vi "SR830Test.vi"() -> ()   [LabVIEW 2013]
uses:
  <vilib>/Instr/_visa.llb/VISA Configure Serial Port (Instr).vi
panel:
  out "read buffer":string
  in  "VISA resource name":refnum<visa-resource-name>
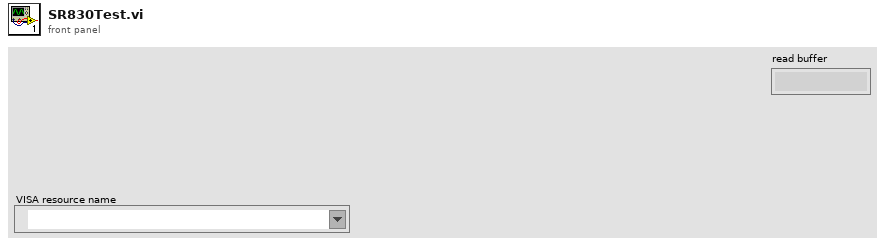
[diagram p1: front panel]
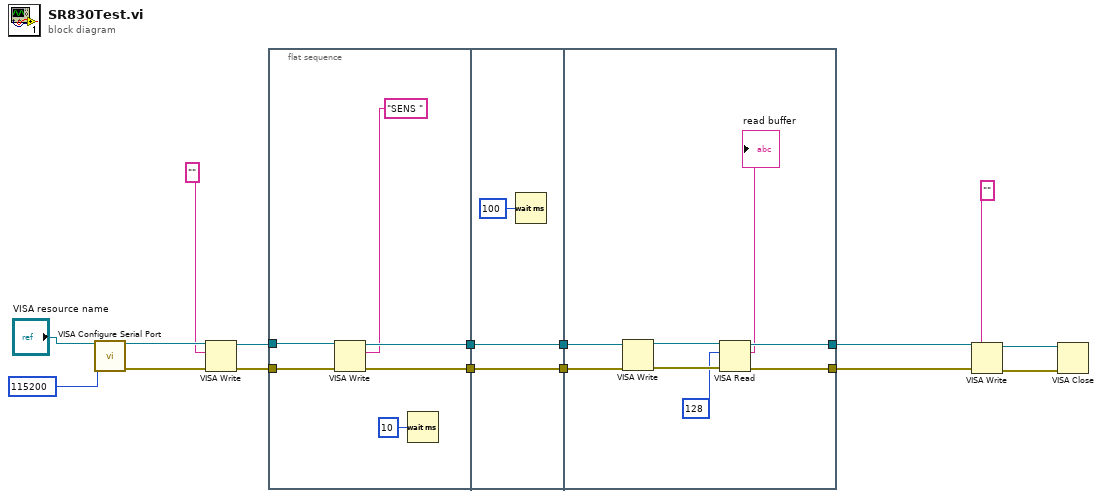
[diagram p0: block diagram]
diagram:
  n1 = call-poly "VISA Configure Serial Port"("VISA resource name"="VISA resource name", "baud rate (9600)"=u32 115200) -> ("VISA resource name out"=w12:refnum<visa-resource-name>, "error out"=w10:errorcluster)  [unwired: 12 in]
  n2 = VISA Write(VISA resource name=w12, write buffer="", error in (no error)=w10) -> (VISA resource name out=w11:refnum<visa-resource-name>, error out=w9:errorcluster)  [unwired: 1 out]
  n3 = flat-sequence {
    tunnel: w11 -> [w22]
    tunnel: w9 -> [w21]
    tunnel: [w20] -> w14
    tunnel: [w19] -> w13
    tunnel: w14 -> [w24]
    tunnel: w13 -> [w23]
    tunnel: [w24] -> w8
    tunnel: [w23] -> w7
    tunnel: w8 -> [w33]
    tunnel: w7 -> [w32]
    tunnel: [w29] -> w6
    tunnel: [w28] -> w5
    frame #0 {
      n4 = VISA Write(VISA resource name=w22, write buffer="SENS ", error in (no error)=w21) -> (VISA resource name out=w20:refnum<visa-resource-name>, error out=w19:errorcluster)  [unwired: 1 out]
      n5 = Wait (ms)(milliseconds to wait=u32 10) -> ()  [unwired: 1 out]
    }
    frame #1 {
      n6 = Wait (ms)(milliseconds to wait=u32 100) -> ()  [unwired: 1 out]
    }
    frame #2 {
      n7 = VISA Write(VISA resource name=w33, error in (no error)=w32) -> (VISA resource name out=w31:refnum<visa-resource-name>, error out=w30:errorcluster)  [unwired: 1 in, 1 out]
      n8 = VISA Read(VISA resource name=w31, byte count=u32 128, error in (no error)=w30) -> (VISA resource name out=w29:refnum<visa-resource-name>, read buffer=→"read buffer":string, error out=w28:errorcluster)  [unwired: 1 out]
    }
  }
  n9 = VISA Write(VISA resource name=w6, write buffer="", error in (no error)=w5) -> (VISA resource name out=w4:refnum<visa-resource-name>, error out=w3:errorcluster)  [unwired: 1 out]
  n10 = VISA Close(VISA resource name=w4, error in (no error)=w3) -> ()  [unwired: 1 out]
